vi "Find Record By Account.vi"(8 "error in":errorcluster, 11 "Account Number":i32) -> (0 "error out":errorcluster, 3 "DB Item":T1 {"Balance" format="%#.2g"})   [LabVIEW 2020, in "Configuration Database.lvlib"]
doc: "Internal Reference holder for Database"
uses:
  Configuration Database.lvlib
  Controls/DB item.ctl
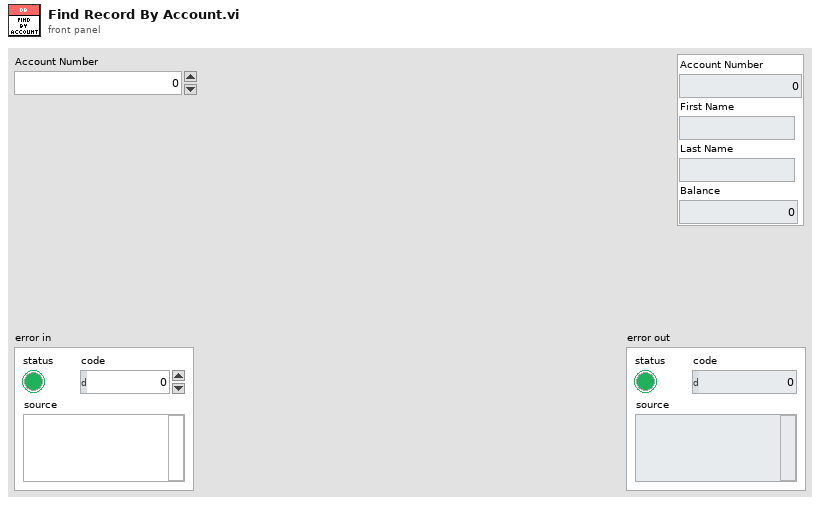
[diagram p1: front panel]
types:
  T1 = typedef "Configuration Database.lvlib/DB item.ctl" = cluster{"Account Number":i32, "First Name":string, "Last Name":string, "Balance":dbl}
  T2 = typedef "Configuration Database.lvlib/FGV Data.ctl" = cluster{"CSV File Path":path, "Records":T1[]}
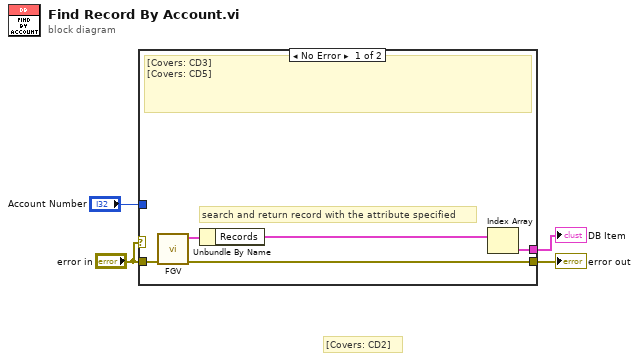
[diagram p0: block diagram]
diagram:
  # "[Covers: CD2]"
  n1 = case shown="No Error" "error in" {
    tunnel: [w8 w10] -> w4
    tunnel: "error in" -> [w9 w10]
    tunnel: [w5 _] -> w2
    tunnel: "Account Number" -> [_ _]
    frame No Error {
      # "search and return record with the attribute specified"
      # "[Covers: CD3]\n[Covers: CD5]"
      n2 = call "FGV.vi"("error in"=w9) -> ("error out"=w8:errorcluster, "Defaults"=w7:T2)  [unwired: 9 in]
      n3 = Unbundle By Name(w7) -> ("Records"=w6:T1[])
      n4 = Index Array(array=w6) -> (element=w5:T1)  [unwired: 1 in]
    }
    frame Error {
    }
  }
  "error out" <- w4
  "DB Item" <- w2
